vi "update.vi"(8 "error in (no error)":errorcluster, 11 "ColorOverlay in":refnum<class "ColorOverlay.lvclass">) -> (0 "error out":errorcluster, 2 "color cluster out":cluster{"Red":u8, "Green":u8, "Blue":u8}[](array[cluster]), 3 "ColorOverlay out":refnum<class "ColorOverlay.lvclass">)   [LabVIEW 2010, in "ColorOverlay.lvclass"]
uses:
  ColorOverlay.lvclass
  ColorOverlay.lvclass/ColorOverlay.ctl
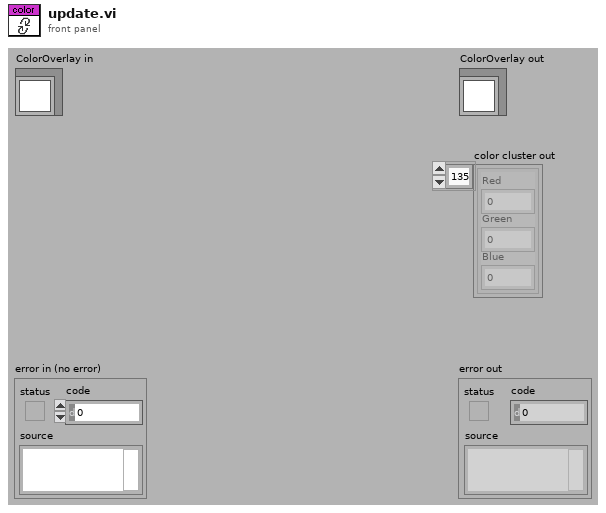
[diagram p1: front panel]
types:
  T1 = cluster{"Numeric":u32, "Numeric":u32, "Numeric":u32}[]
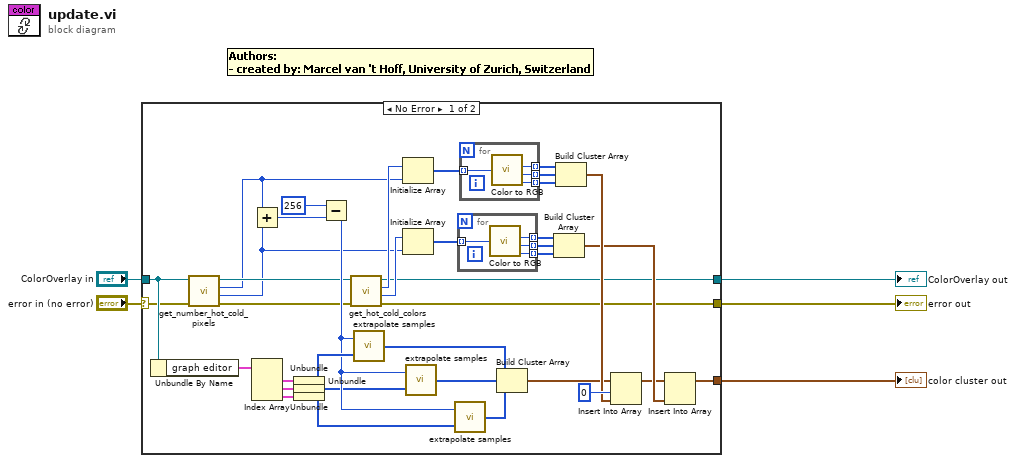
[diagram p0: block diagram]
diagram:
  n1 = case shown="No Error" "error in (no error)" {
    selector: "error in (no error)" -> [w12 w52]
    tunnel: [w8 w52] -> w4
    tunnel: [w7 w51] -> w2
    tunnel: "ColorOverlay in" -> [w14 w51]
    tunnel: [w6 _] -> w1
    frame No Error {
      n2 = Unbundle By Name(w14) -> ("graph editor"=w42:cluster{"ramp array out":u32[]}[])
      n3 = call-dynamic "get_number_hot_cold_pixels.vi"("error in (no error)"=w12, "ColorOverlay in"=w14) -> ("error out"=w11:errorcluster, "# hot pixels"=w9:i32, "# cold pixels"=w10:i32, "ColorOverlay out"=w13:refnum<class "ColorOverlay.lvclass">)  [unwired: 6 in]
      n4 = Add(x=w10, y=w9) -> (x+y=w36:i32)
      n5 = Index Array(array=w42) -> (element #1=w41:cluster{"ramp array out":u32[]}, element #2=w39:cluster{"ramp array out":u32[]}, element #3=w38:cluster{"ramp array out":u32[]})  [unwired: 3 in]
      n6 = Unbundle(w41) -> ("ramp array out"=w40:u32[])
      n7 = Unbundle(w39) -> ("ramp array out"=w34:u32[])
      n8 = Unbundle(w38) -> ("ramp array out"=w33:u32[])
      n9 = Subtract(x=256, y=w36) -> (x-y=w35:i32)
      n10 = call-dynamic "get_hot_cold_colors.vi"("error in (no error)"=w11, "ColorOverlay in"=w13) -> ("error out"=w8:errorcluster, "color upper limit"=w15:u32, "color lower limit"=w16:u32, "ColorOverlay out"=w7:refnum<class "ColorOverlay.lvclass">)  [unwired: 6 in]
      n11 = call "extrapolate samples.vi"("ramp array in"=w40, "new sample number"=w35) -> ("extrapolated array out"=w32:u32[])
      n12 = Initialize Array(w16, w10) -> (w20:u32[])
      n13 = Initialize Array(w15, w9) -> (w28:u32[])
      n14 = call "extrapolate samples.vi"("ramp array in"=w34, "new sample number"=w35) -> ("extrapolated array out"=w31:u32[])
      n15 = call "extrapolate samples.vi"("ramp array in"=w33, "new sample number"=w35) -> ("extrapolated array out"=w30:u32[])
      n16 = for {
        tunnel: w28 -> [w46] mode=indexing
        tunnel: [w45] -> w27 mode=indexing
        tunnel: [w44] -> w26 mode=indexing
        tunnel: [w43] -> w25 mode=indexing
        n17 = call <vilib>:"Color to RGB.vi"("Color"=w46) -> ("R"=w45:u8, "G"=w44:u8, "B"=w43:u8)  [unwired: 1 out]
      }
      n18 = for {
        tunnel: w20 -> [w50] mode=indexing
        tunnel: [w49] -> w21 mode=indexing
        tunnel: [w48] -> w22 mode=indexing
        tunnel: [w47] -> w23 mode=indexing
        n19 = call <vilib>:"Color to RGB.vi"("Color"=w50) -> ("R"=w49:u8, "G"=w48:u8, "B"=w47:u8)  [unwired: 1 out]
      }
      n20 = Build Cluster Array(w32, w31, w30) -> (w17:T1)
      n21 = Build Cluster Array(w27, w26, w25) -> (w19:cluster{"R":u8, "G":u8, "B":u8}[])
      n22 = Build Cluster Array(w21, w22, w23) -> (w24:cluster{"R":u8, "G":u8, "B":u8}[])
      n23 = Insert Into Array(array=w17, index=0, new element=w24) -> (w18:T1)
      n24 = Insert Into Array(array=w18, new element=w19) -> (w6:T1)  [unwired: 1 in]
    }
    frame Error {
    }
  }
  "error out" <- w4
  "ColorOverlay out" <- w2
  "color cluster out" <- w1
